vi "Set Label.vi"(8 "error in (no error)":errorcluster, 10 "Label":string, 11 "MMI Scaling in":refnum<class "IObject.lvclass">) -> (0 "error out":errorcluster, 3 "MMI Scaling out":refnum<class "IObject.lvclass">)   [LabVIEW 2013, in "IObject.lvclass"]
uses:
  IObject.lvclass
  IObject.lvclass/IObject.ctl
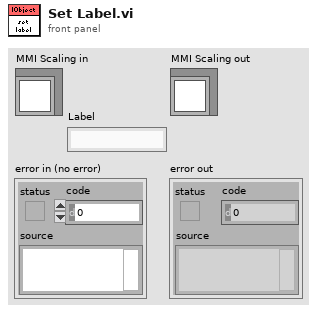
[diagram p1: front panel]
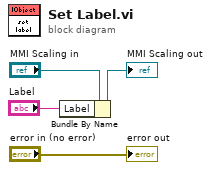
[diagram p0: block diagram]
diagram:
  n1 = Bundle By Name(cluster="MMI Scaling in", "Label"="Label") -> (→"MMI Scaling out":refnum<class "IObject.lvclass">)
  "error out" <- "error in (no error)"
